vi "Solve Linear Eqs (Gen, single right hand).vi"(9 "relative tolerance":dbl=-1.0, 10 "Known Vector":dbl[](array[numeric]), 11 "Input Matrix":T1) -> (0 "error":i32, 3 "Solution Vector":dbl[](array[numeric]))   [LabVIEW 2010, in "NI_AALPro.lvlib"]
uses:
  NI_AALPro.lvlib
  RealMatrix.ctl
  NI_AALBase.lvlib
  NI_Matrix.lvlib
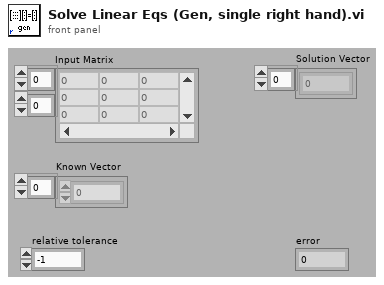
[diagram p1: front panel]
types:
  T1 = typedef "NI_Matrix.lvlib/RealMatrix.ctl" = dbl[][]
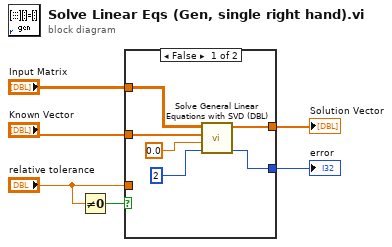
[diagram p0: block diagram]
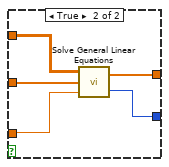
[diagram p2: hidden frame]
diagram:
  n1 = Not Equal To 0?(x="relative tolerance") -> (x != 0?=w6:bool)
  n2 = case shown="False" w6 {
    tunnel: "relative tolerance" -> [_ w17]
    tunnel: "Known Vector" -> [w11 w16]
    tunnel: "Input Matrix" -> [w12 w15]
    tunnel: [w7 w14] -> w2
    tunnel: [w8 w13] -> w1
    frame False {
      n3 = call "Solve General Linear Equations with SVD (DBL).vi"("iteration"=2, "relative tolerance"=0.0, "Known Vector"=w11, "Input Matrix"=w12) -> ("error"=w7:i32, "Solution Vector"=w8:dbl[])  [unwired: 6 in]
    }
    frame True {
      n4 = call "Solve General Linear Equations.vi"("relative tolerance"=w17, "Known Vector"=w16, "Input Matrix"=w15) -> ("error"=w14:i32, "Solution Vector"=w13:dbl[])
    }
  }
  "Solution Vector" <- w1
  "error" <- w2
